vi "Initialize Active Options.vi"(8 "error in (no error)":errorcluster, 11 "Normal Active Option View in":refnum<class "Normal Active Option View.lvclass">) -> (0 "error out":errorcluster, 3 "Normal Active Option View out":refnum<class "Normal Active Option View.lvclass">)   [LabVIEW 2019, in "Normal Active Option View.lvclass"]
uses:
  <vilib>/gpm_packages/@cs/Car-wash/Source/Normal Active Station View/Normal Active Station View/Normal Active Option View.lvclass
  <vilib>/gpm_packages/@cs/Car-wash/Source/Normal Active Station View/Normal Active Station View/Normal Active Option View.lvclass/Normal Active Option View.ctl
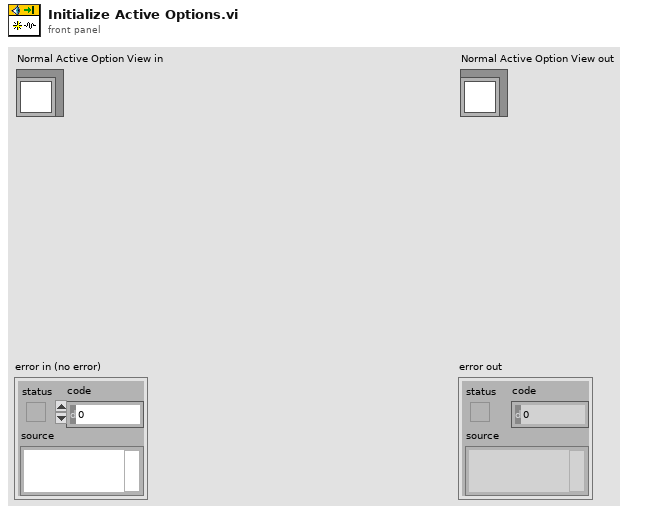
[diagram p1: front panel]
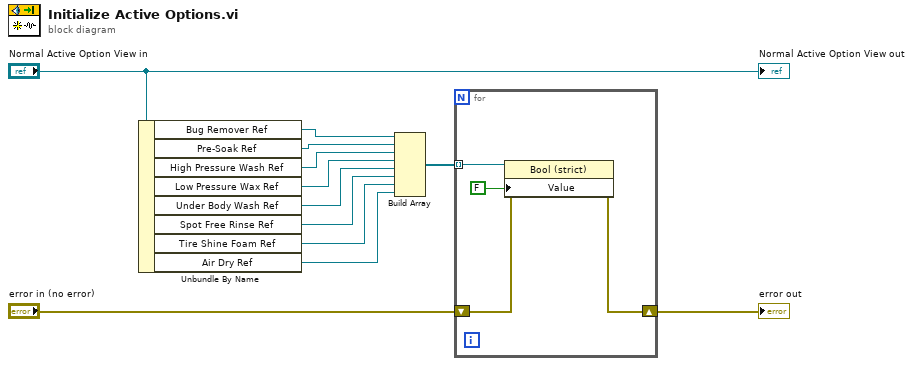
[diagram p0: block diagram]
diagram:
  n1 = Unbundle By Name("Normal Active Option View in") -> ("Bug Remover Ref"=w11:refnum<vi>, "Pre-Soak Ref"=w10:refnum<vi>, "High Pressure Wash Ref"=w9:refnum<vi>, "Low Pressure Wax Ref"=w8:refnum<vi>, "Under Body Wash Ref"=w7:refnum<vi>, "Spot Free Rinse Ref"=w6:refnum<vi>, "Tire Shine Foam Ref"=w5:refnum<vi>, "Air Dry Ref"=w4:refnum<vi>)
  n2 = Build Array(w11, w10, w9, w8, w7, w6, w5, w4) -> (w1:refnum<vi>[])
  n3 = for {
    shift-right: [w14] -> w2
    shift-left: "error in (no error)" -> [w15]
    tunnel: w1 -> [w16] mode=indexing
    n4 = property class="Bool (strict)"(reference=w16, error in=w15, "Value"=FALSE) -> (error out=w14:errorcluster)  [unwired: 1 out]
  }
  "error out" <- w2
  "Normal Active Option View out" <- "Normal Active Option View in"
